vi "Vector3D to Array.vi"(1 "Vector3D":T1={"Thumb"=[0.0, 0.0, 0.0], "Middle"=[0.0, 0.0, 0.0], "Index"=[0.0, 0.0, 0.0]}) -> (0 "Array":dbl[](array[numeric]))   [LabVIEW 2011]
uses:
  Controls/Vector3D Fingers.ctl
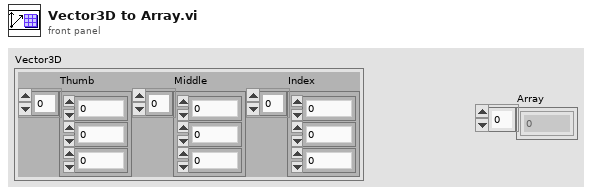
[diagram p1: front panel]
types:
  T1 = typedef "Vector3D Fingers.ctl" = cluster{"Thumb":dbl[], "Middle":dbl[], "Index":dbl[]}
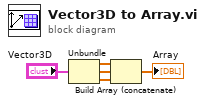
[diagram p0: block diagram]
diagram:
  n1 = Unbundle("Vector3D") -> ("Thumb"=w4:dbl[], "Middle"=w3:dbl[], "Index"=w2:dbl[])
  n2 = Build Array (concatenate)(w4, w3, w2) -> (→"Array":dbl[])
